vi "读取PLC数据信息 .vi"(11 "PLC原始IO数据":string) -> (0 "子数组":bool[](array[boolean]))   [LabVIEW 2011]
panel:
  out "长度":i32
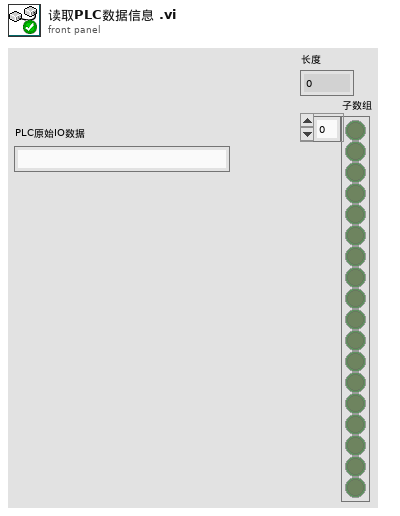
[diagram p1: front panel]
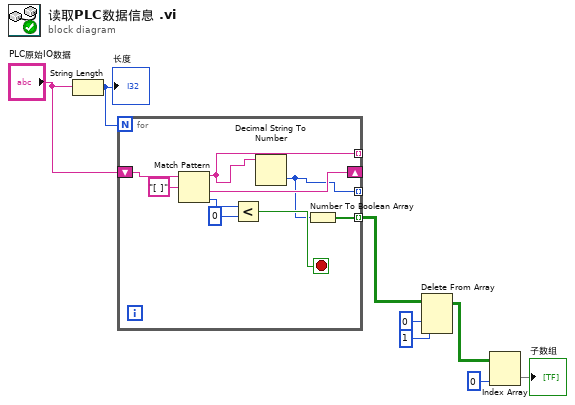
[diagram p0: block diagram]
diagram:
  n1 = String Length(string="PLC原始IO数据") -> (length=w8:i32)
  "长度" <- w8
  n2 = for {
    N: w8 -> [_]
    shift-right: [w12] -> _
    shift-left: "PLC原始IO数据" -> [w17]
    tunnel: [w10] -> _ mode=indexing
    tunnel: [w11] -> _ mode=indexing
    tunnel: [w9] -> w4 mode=indexing
    stop <- w13 stop-if-true
    n3 = Match Pattern(string=w17, regular expression="[ ]" ("正则表达式")) -> (before substring=w11:string, after substring=w12:string, offset past match=w15:i32)  [unwired: 1 in, 1 out]
    n4 = Less?(x=w15, y=0) -> (x < y?=w13:bool)
    n5 = Decimal String To Number(string=w11) -> (number=w10:i32)  [unwired: 2 in, 1 out]
    n6 = Number To Boolean Array(number=w10) -> (Boolean array=w9:bool[])
  }
  n7 = Delete From Array(array=w4, length=1 ("长度"), index (row)=0 ("索引 (行)")) -> (array with subset deleted=w3:bool[][])  [unwired: 1 in, 1 out]
  n8 = Index Array(array=w3, index (col)=0 ("禁用的索引 (列)")) -> (element=→"子数组":bool[])  [unwired: 1 in]
